vi "VI Tree.vi"   [LabVIEW 2013, in "SRS SR400.lvlib"]
uses:
  <instrlib>/SRS SR400/SRS SR400.lvlib
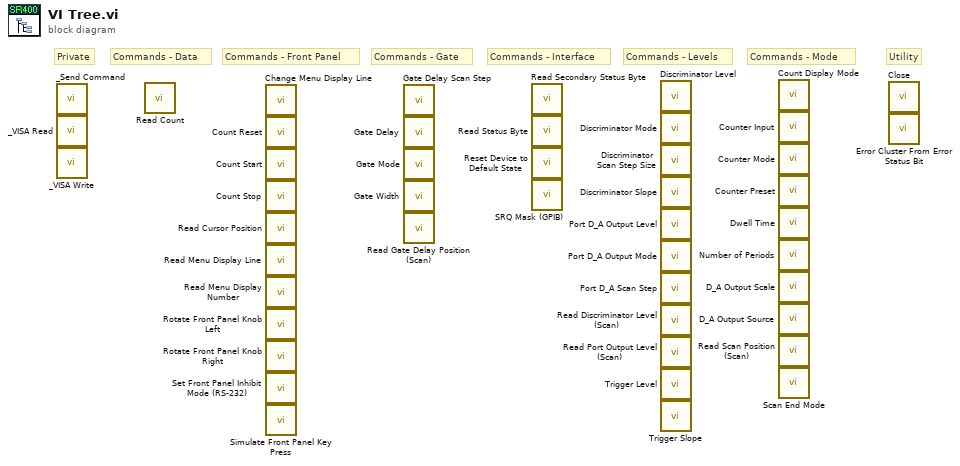
[diagram p0: block diagram]
diagram:
  # "Utility"
  # "Commands - Data"
  # "Commands - Mode"
  # "Commands - Levels"
  # "Private"
  # "Commands - Interface"
  # "Commands - Gate"
  # "Commands - Front Panel"
  n1 = call <instrlib>:"_Send Command.vi"() -> ()  [unwired: 9 in, 3 out]
  n2 = call <instrlib>:"_VISA Read.vi"() -> ()  [unwired: 9 in, 3 out]
  n3 = call <instrlib>:"_VISA Write.vi"() -> ()  [unwired: 10 in, 2 out]
  n4 = call <instrlib>:"Read Count.vi"() -> ()  [unwired: 9 in, 3 out]
  n5 = call <instrlib>:"Change Menu Display Line.vi"() -> ()  [unwired: 10 in, 2 out]
  n6 = call <instrlib>:"Count Reset.vi"() -> ()  [unwired: 10 in, 2 out]
  n7 = call <instrlib>:"Count Start.vi"() -> ()  [unwired: 10 in, 2 out]
  n8 = call <instrlib>:"Count Stop.vi"() -> ()  [unwired: 10 in, 2 out]
  n9 = call <instrlib>:"Read Cursor Position.vi"() -> ()  [unwired: 9 in, 3 out]
  n10 = call <instrlib>:"Read Menu Display Line.vi"() -> ()  [unwired: 9 in, 3 out]
  n11 = call <instrlib>:"Read Menu Display Number.vi"() -> ()  [unwired: 9 in, 3 out]
  n12 = call <instrlib>:"Rotate Front Panel Knob Left.vi"() -> ()  [unwired: 10 in, 2 out]
  n13 = call <instrlib>:"Rotate Front Panel Knob Right.vi"() -> ()  [unwired: 10 in, 2 out]
  n14 = call <instrlib>:"Set Front Panel Inhibit Mode (RS-232).vi"() -> ()  [unwired: 10 in, 2 out]
  n15 = call <instrlib>:"Simulate Front Panel Key Press.vi"() -> ()  [unwired: 10 in, 2 out]
  n16 = call <instrlib>:"Gate Delay Scan Step.vi"() -> ()  [unwired: 9 in, 3 out]
  n17 = call <instrlib>:"Gate Delay.vi"() -> ()  [unwired: 9 in, 3 out]
  n18 = call <instrlib>:"Gate Mode.vi"() -> ()  [unwired: 9 in, 3 out]
  n19 = call <instrlib>:"Gate Width.vi"() -> ()  [unwired: 9 in, 3 out]
  n20 = call <instrlib>:"Read Gate Delay Position (Scan).vi"() -> ()  [unwired: 9 in, 3 out]
  n21 = call <instrlib>:"Read Secondary Status Byte.vi"() -> ()  [unwired: 8 in, 4 out]
  n22 = call <instrlib>:"Read Status Byte.vi"() -> ()  [unwired: 8 in, 4 out]
  n23 = call <instrlib>:"Reset Device to Default State.vi"() -> ()  [unwired: 10 in, 2 out]
  n24 = call <instrlib>:"SRQ Mask (GPIB).vi"() -> ()  [unwired: 9 in, 3 out]
  n25 = call <instrlib>:"Discriminator Level.vi"() -> ()  [unwired: 9 in, 3 out]
  n26 = call <instrlib>:"Discriminator Mode.vi"() -> ()  [unwired: 9 in, 3 out]
  n27 = call <instrlib>:"Discriminator Scan Step Size.vi"() -> ()  [unwired: 9 in, 3 out]
  n28 = call <instrlib>:"Discriminator Slope.vi"() -> ()  [unwired: 9 in, 3 out]
  n29 = call <instrlib>:"Port D_A Output Level.vi"() -> ()  [unwired: 9 in, 3 out]
  n30 = call <instrlib>:"Port D_A Output Mode.vi"() -> ()  [unwired: 9 in, 3 out]
  n31 = call <instrlib>:"Port D_A Scan Step.vi"() -> ()  [unwired: 9 in, 3 out]
  n32 = call <instrlib>:"Read Discriminator Level (Scan).vi"() -> ()  [unwired: 9 in, 3 out]
  n33 = call <instrlib>:"Read Port Output Level (Scan).vi"() -> ()  [unwired: 9 in, 3 out]
  n34 = call <instrlib>:"Trigger Level.vi"() -> ()  [unwired: 9 in, 3 out]
  n35 = call <instrlib>:"Trigger Slope.vi"() -> ()  [unwired: 9 in, 3 out]
  n36 = call <instrlib>:"Count Display Mode.vi"() -> ()  [unwired: 9 in, 3 out]
  n37 = call <instrlib>:"Counter Input.vi"() -> ()  [unwired: 9 in, 3 out]
  n38 = call <instrlib>:"Counter Mode.vi"() -> ()  [unwired: 9 in, 3 out]
  n39 = call <instrlib>:"Counter Preset.vi"() -> ()  [unwired: 9 in, 3 out]
  n40 = call <instrlib>:"Dwell Time.vi"() -> ()  [unwired: 9 in, 3 out]
  n41 = call <instrlib>:"Number of Periods.vi"() -> ()  [unwired: 9 in, 3 out]
  n42 = call <instrlib>:"D_A Output Scale.vi"() -> ()  [unwired: 9 in, 3 out]
  n43 = call <instrlib>:"D_A Output Source.vi"() -> ()  [unwired: 9 in, 3 out]
  n44 = call <instrlib>:"Read Scan Position (Scan).vi"() -> ()  [unwired: 9 in, 3 out]
  n45 = call <instrlib>:"Scan End Mode.vi"() -> ()  [unwired: 9 in, 3 out]
  n46 = call <instrlib>:"Close.vi"() -> ()  [unwired: 11 in, 1 out]
  n47 = call <instrlib>:"Error Cluster From Error Status Bit.vi"() -> ()  [unwired: 10 in, 2 out]
